vi "CoreTestHarness.vi"() -> ()   [LabVIEW 2017]
uses:
  Interface/Configuration.ctl
  <vilib>/rvi/Analysis/control/PID/Typedef/niFpgaPID_PIGains.ctl
  <vilib>/rvi/Analysis/control/PID/Typedef/niFpgaPID_OutputRange.ctl
  FPGA/HarmonicFilter.ctl
  <instrlib>/_niInstr/FIFO Register Bus/v1/Host/niInstr FIFO Register Bus v1 Host.lvclass
  C:/Program Files (x86)/National Instruments/LabVIEW 2017/instr.lib/_niInstr/Instruction Framework/v1/Host/Instruction Target/niInstr Instruction Target v1 Host.lvclass
  <vilib>/FPGAPlugInAG/sbRIO-9607/niLvFpga_Open_sbRIO-9607.vi
  <vilib>/rvi/interface/common/dynamic/niFpgaDynamicAddResources.vi
  <vilib>/FPGAPlugInAG/Dynamic/niLvFpga_Reset_Dynamic.vi
  <vilib>/rvi/interface/common/niFpgaWaitOnOcc.vi
  <vilib>/Utility/error.llb/Error Cluster From Error Code.vi
  <vilib>/rvi/errors/niLvFpgaAdjustHostInterfaceError.vi
  <vilib>/FPGAPlugInAG/Dynamic/niLvFpga_Run_Dynamic.vi
  <vilib>/rvi/interface/nirviOpenFPGA/nirviOpenFPGA.xnode
  FPGA Bitfiles/ThreePhasePLLdev_FPGATarget_ThreePhasePLLdev_cNgKxiCEvCc.lvbitx
  FPGA/ThreePhasePLL_dev.vi
  <vilib>/rvi/interface/nirviMethod/nirviMethod.xnode
  <vilib>/rvi/interface/nirviReadWriteControl/nirviReadWriteControl.xnode
  Interface/ThreePhasePLLInterface.lvlib
  <vilib>/rvi/interface/Simulation/niFpgaSimulationCallBeginRW.vi
  NiFpgaLv.dll
  <vilib>/FPGAPlugInAG/Dynamic/niLvFpga_ConfigureFifo_Dynamic.vi
  <vilib>/rvi/errors/niLvFpgaMergeErrorWithErrorCode.vi
  <vilib>/FPGAPlugInAG/Dynamic/niLvFpga_StartFifo_Dynamic.vi
  <vilib>/FPGAPlugInAG/Dynamic/niLvFpga_ReadFifo_Dynamic.vi
  FPGA/ThreePhasePLL.lvlib
panel:
  in  "GenFreqRadPerSec":sgl
  out "Waveforms":sgl[][](graph)
  out "PLLTimingActual":u32
  out "ThreePhaseGenActual":u32
  out "theta error":sgl
  out "freq error":sgl
  in  "reset":bool
  out "detectedFreq":sgl
  out "Locked":bool
  in  "Configuration":T1={"PLLgains"={"proportional gain"=100.0, "integral gain"=1e-05}, "PLLrange"={"output high (Inf)"=inf, "output low (-Inf)"=0.0}, "dT"=1e-05, "expectedFreq"=376.911, "lockDuration"=3.0, "freqBoundaries"=1.0, "adjustTheta"=0.015079, "HarmonicFilter"={"enable"=TRUE, "coeff"={"ak"=-0.994986, "bk"=0.00250698}}} {"PLLgains"."proportional gain" step=0.125}
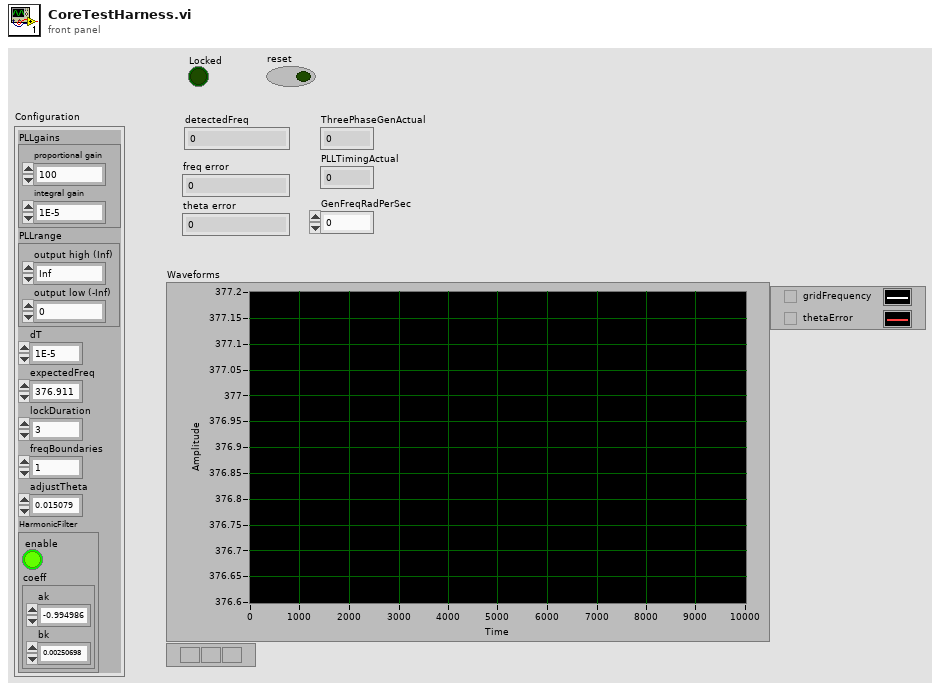
[diagram p1: front panel]
types:
  T1 = typedef "ThreePhasePLLInterface.lvlib/Configuration.ctl" = cluster{"PLLgains":T2, "PLLrange":T3, "dT":sgl, "expectedFreq":sgl, "lockDuration":sgl, "freqBoundaries":sgl, "adjustTheta":sgl, "HarmonicFilter":cluster{"enable":bool, "coeff":T4}}
  T2 = typedef "niFpgaPID_PIGains.ctl" = cluster{"proportional gain":sgl, "integral gain":sgl}
  T3 = typedef "niFpgaPID_OutputRange.ctl" = cluster{"output high (Inf)":sgl, "output low (-Inf)":sgl}
  T4 = typedef "ThreePhasePLL.lvlib/HarmonicFilter.ctl" = cluster{"ak":sgl, "bk":sgl}
  T5 = typedef "ThreePhasePLLInterface.lvlib/InterfaceRef.ctl" = cluster{"instruction target":refnum<class "niInstr Instruction Target v1 Host.lvclass">, "context":refnum<class "niInstr Instruction Framework Context v1 Host.lvclass">}
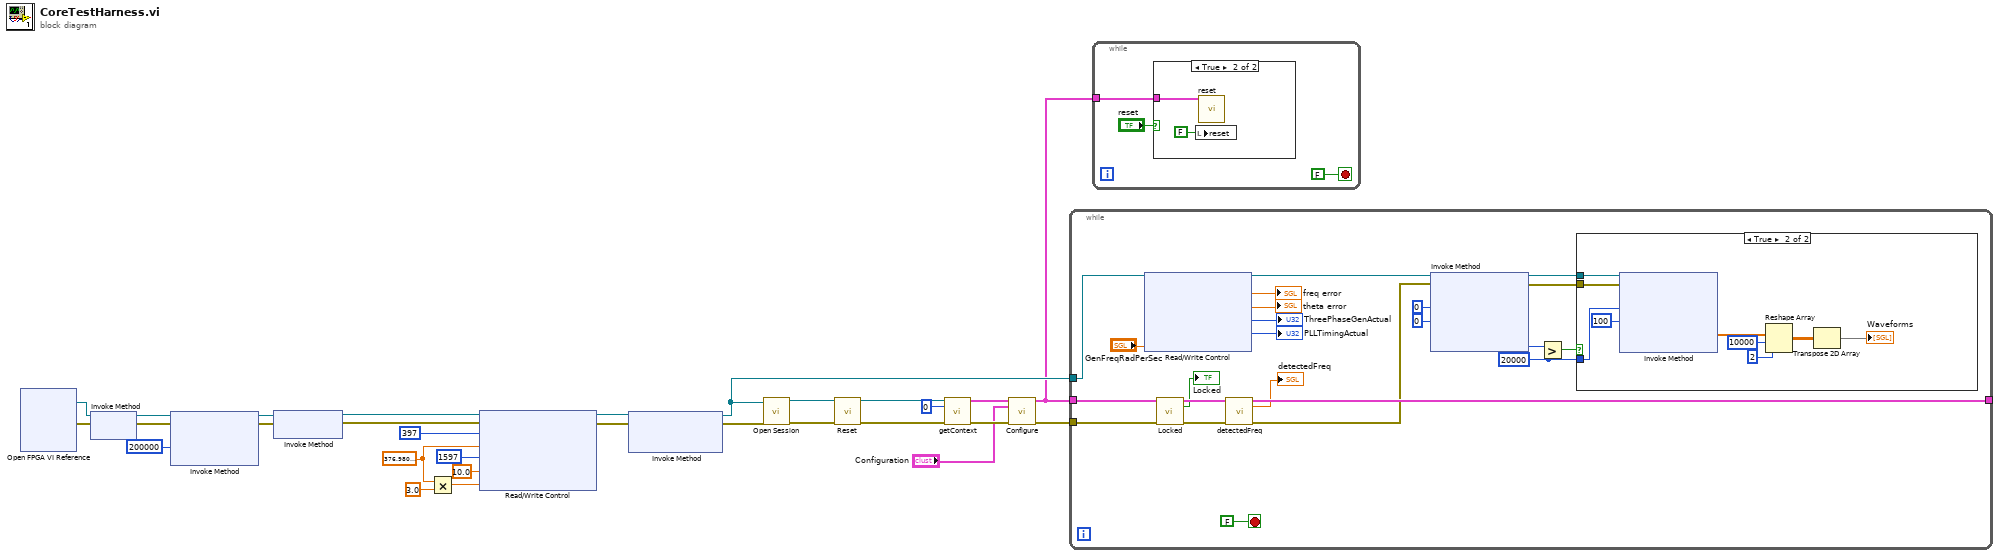
[diagram p0: block diagram]
diagram:
  w10 = sgl 376.98 ("GenFreqRadPerSec")
  n1 = xnode "Open FPGA VI Reference"() -> ("FPGA VI Reference Out"=w17:refnum<k20>, "error out"=w18:errorcluster)  [unwired: 2 in]
  n2 = xnode "Invoke Method"("FPGA VI Reference In"=w17, "error in"=w18) -> ("FPGA VI Reference Out"=w8:refnum<k20>, "error out"=w7:errorcluster)
  n3 = xnode "Invoke Method"("FPGA VI Reference In"=w8, "error in"=w7, "Requested Depth"=u32 200000) -> ("FPGA VI Reference Out"=w5:refnum<k20>, "error out"=w4:errorcluster)  [unwired: 1 out]
  n4 = xnode "Invoke Method"("FPGA VI Reference In"=w5, "error in"=w4) -> ("FPGA VI Reference Out"=w3:refnum<k20>, "error out"=w2:errorcluster)
  n5 = Multiply(x=w10, y=sgl 3.0) -> (x*y=w11:sgl)
  n6 = xnode "Read/Write Control"("FPGA VI Reference In"=w3, "error in"=w2, "ThreePhaseGenTiming"=u32 397, "GenFreqRadPerSec"=w10, "PLL_Timing"=u32 1597, "HarmonicGain"=sgl 10.0, "HarmonicFreqRadPerSec"=w11) -> ("FPGA VI Reference Out"=w15:refnum<k20>, "error out"=w14:errorcluster)
  n7 = xnode "Invoke Method"("FPGA VI Reference In"=w15, "error in"=w14) -> ("FPGA VI Reference Out"=w21:refnum<k20>, "error out"=w27:errorcluster)  [unwired: 1 in]
  n8 = call <instrlib>:"Open Session.vi"("fpga ref"=w21, "error in"=w27) -> ("session out"=w28:refnum<class "niInstr FIFO Register Bus v1 Host.lvclass">, "error out"=w29:errorcluster)  [unwired: 12 in]
  n9 = call-dynamic "Reset.vi"("session in"=w28, "error in"=w29) -> ("session out"=w26:refnum<class "niInstr FIFO Register Bus v1 Host.lvclass">, "error out"=w25:errorcluster)  [unwired: 12 in]
  n10 = call "getContext.vi"("instruction target in"=w26, "instance"=u8 0, "error in"=w25) -> ("Interface"=w23:T5, "error out"=w22:errorcluster)  [unwired: 11 in]
  n11 = call "Configure.vi"("Interface in"=w23, "Configuration"="Configuration", "error in"=w22) -> ("Interface out"=w16:T5, "error out"=w20:errorcluster)  [unwired: 11 in]
  n12 = while {
    tunnel: w21 -> [w44]
    tunnel: w20 -> [w49]
    tunnel: w16 -> [w48]
    tunnel: [w47] -> _
    stop <- FALSE stop-if-true
    w31 = u32 20000 ("y")
    n13 = xnode "Read/Write Control"("FPGA VI Reference In"=w44, "GenFreqRadPerSec"="GenFreqRadPerSec") -> ("FPGA VI Reference Out"=w39:refnum<k20>, "freq error"=→"freq error":sgl, "theta error"=→"theta error":sgl, "ThreePhaseGenActual"=→"ThreePhaseGenActual":u32, "PLLTimingActual"=→"PLLTimingActual":u32)  [unwired: 1 in, 1 out]
    n14 = call "Locked.vi"("Interface in"=w48, "error in"=w49) -> ("Interface out"=w51:T5, "Locked"=→"Locked":bool, "error out"=w50:errorcluster)  [unwired: 11 in]
    n15 = call "detectedFreq.vi"("Interface in"=w51, "error in"=w50) -> ("Interface out"=w47:T5, "detectedFreq"=→"detectedFreq":sgl, "error out"=w36:errorcluster)  [unwired: 11 in]
    n16 = xnode "Invoke Method"("FPGA VI Reference In"=w39, "error in"=w36, "Number of Elements"=u32 0, "Timeout (ms)"=0) -> ("FPGA VI Reference Out"=w33:refnum<k20>, "error out"=w32:errorcluster, "Elements Remaining"=w35:u32)  [unwired: 1 out]
    n17 = Greater?(x=w35, y=w31) -> (0:w34:bool)
    n18 = case shown="True" w34 {
      tunnel: w33 -> [_ w61]
      tunnel: w32 -> [_ w60]
      tunnel: w31 -> [_ w59]
      frame False {
      }
      frame True {
        n19 = xnode "Invoke Method"("FPGA VI Reference In"=w61, "error in"=w60, "Number of Elements"=w59, "Timeout (ms)"=100) -> ("Data"=w57:sgl[])  [unwired: 3 out]
        n20 = Reshape Array(w57, 10000 ("dimension size"), 2 ("dimension size")) -> (w54:sgl[][])
        n21 = Transpose 2D Array(2D array=w54) -> (transposed array=→"Waveforms":sgl[][])
      }
    }
  }
  n22 = while {
    tunnel: w16 -> [w64]
    stop <- FALSE stop-if-true
    n23 = case shown="True" "reset" {
      tunnel: w64 -> [_ w65]
      frame False {
      }
      frame True {
        n24 = local write "reset"(FALSE ("reset")) -> ()
        n25 = call "reset.vi"("Interface in"=w65) -> ()  [unwired: 13 in, 2 out]
      }
    }
  }
